vi "Compare Lists.vi"(4 "Right List":string, 5 "Left List":string, 6 "Compared Items in":string, 7 "Indent Level in":i32) -> (0 "Decicion Made ?":bool, 1 "In Right Order ?":bool, 2 "Compared Items out":string, 3 "Indent Level out":i32)   [LabVIEW 2020, in "AoC 2022.lvlib"]
uses:
  AoC 2022.lvlib
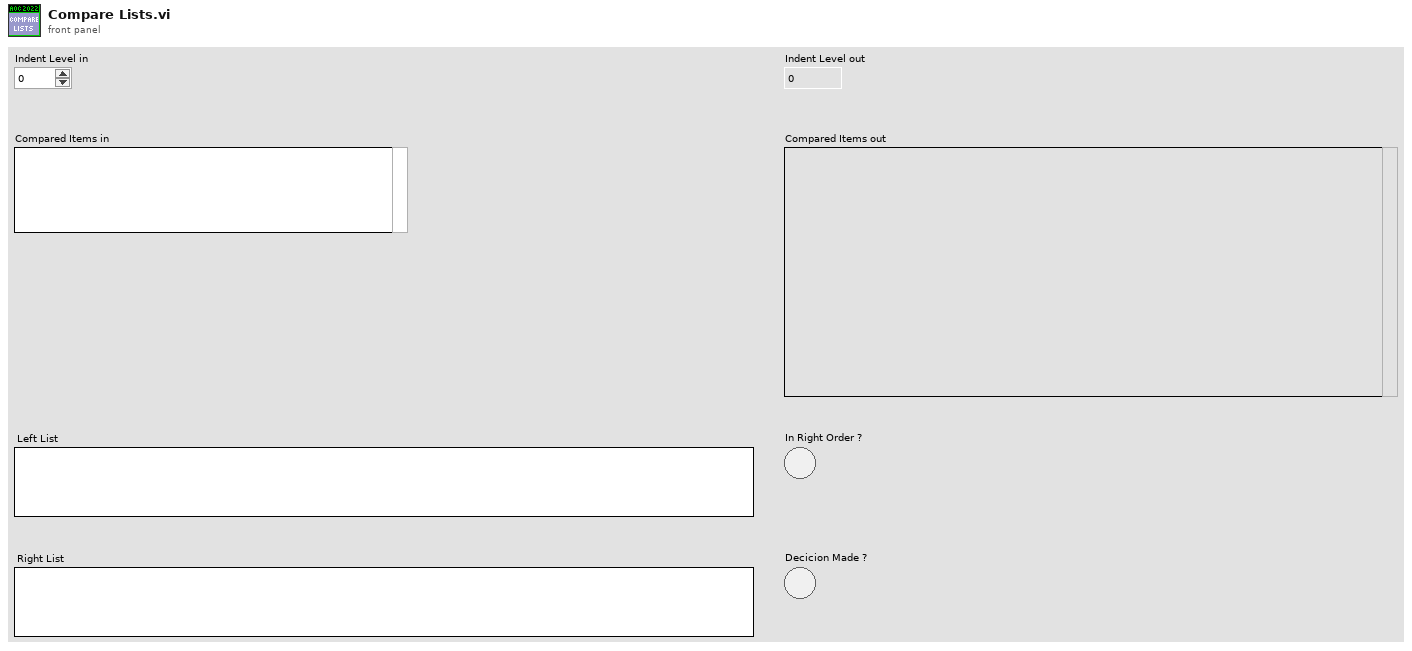
[diagram p1: front panel]
types:
  T1 = typedef "AoC 2022.lvlib/Item.ctl" = cluster{"Item Type":T2, "Item":string}
  T2 = typedef "AoC 2022.lvlib/Item Type.ctl" = enum16{"Integer", "List"}
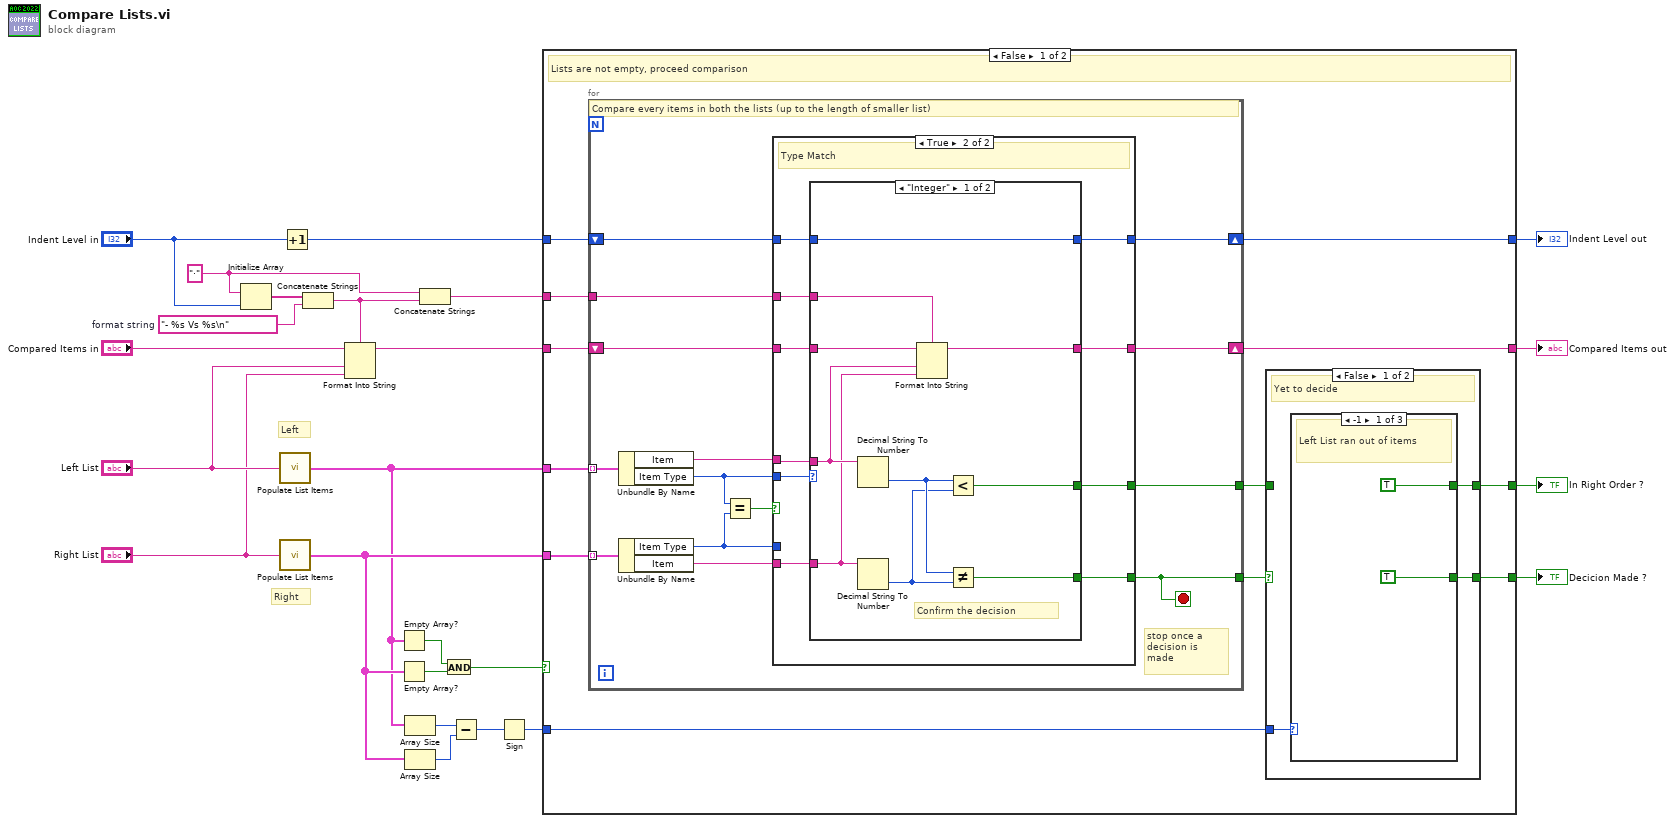
[diagram p0: block diagram]
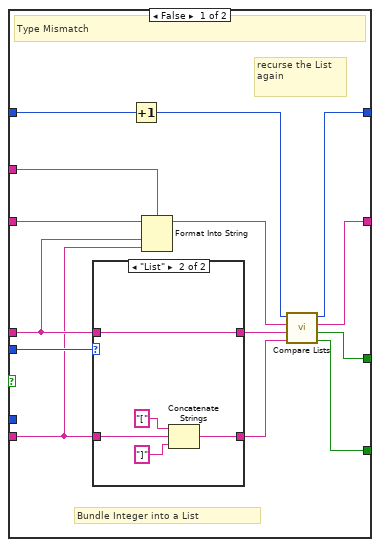
[diagram p2: hidden frame]
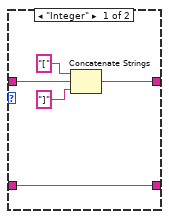
[diagram p3: hidden frame]
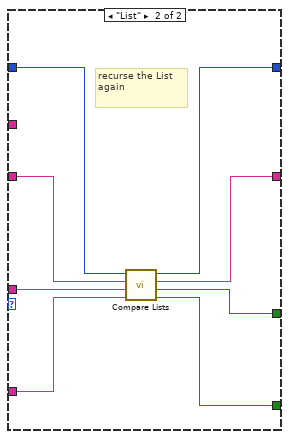
[diagram p4: hidden frame]
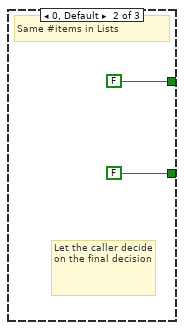
[diagram p5: hidden frame]
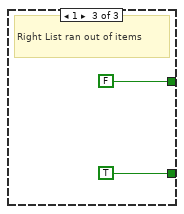
[diagram p6: hidden frame]
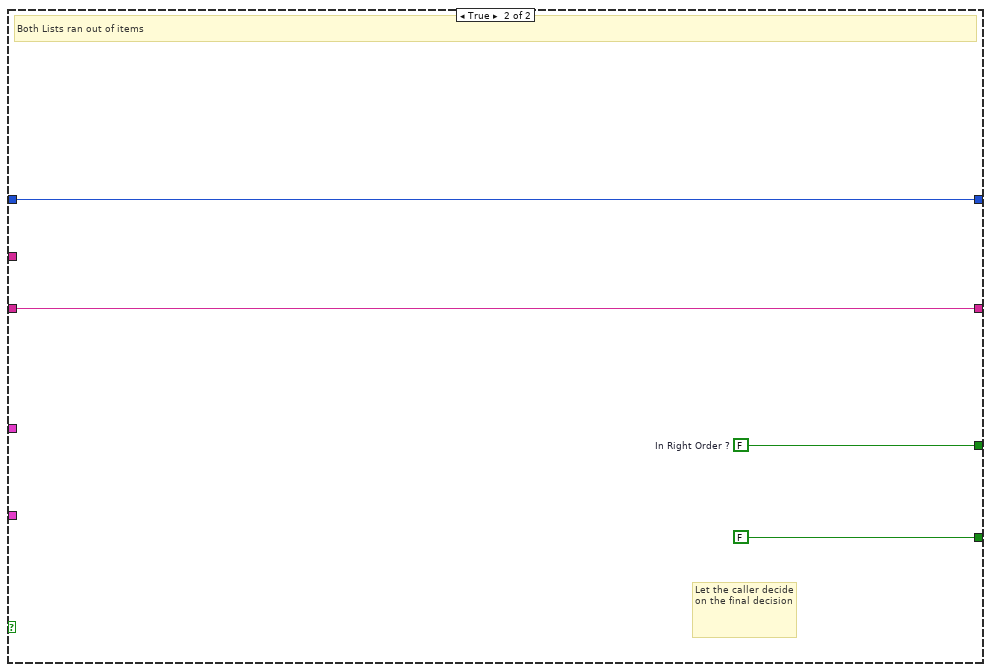
[diagram p8: hidden frame]
diagram:
  w11 = "·"
  w23 = "- %s Vs %s\n"  # format string
  # "Right"
  # "Left"
  n1 = Initialize Array(w11, "Indent Level in") -> (w20:string[])
  n2 = call "Populate List Items.vi"("List"="Left List") -> ("Items"=w8:T1[])
  n3 = call "Populate List Items.vi"("List"="Right List") -> ("Items"=w9:T1[])
  n4 = Increment(x="Indent Level in") -> (x+1=w10:i32)
  n5 = Concatenate Strings(w20, w23) -> (w13:string)
  n6 = Format Into String(format string=w13, initial string="Compared Items in", "Left List", "Right List") -> (resulting string=w16:string)  [unwired: 1 in, 1 out]
  n7 = Empty Array?(array=w8) -> (empty?=w6:bool)
  n8 = Empty Array?(array=w9) -> (empty?=w7:bool)
  n9 = Array Size(array=w8) -> (size(s)=w4:i32)
  n10 = Array Size(array=w9) -> (size(s)=w3:i32)
  n11 = Concatenate Strings(w11, w13) -> (w12:string)
  n12 = And(x=w6, y=w7) -> (x .and. y?=w5:bool)
  n13 = Subtract(x=w4, y=w3) -> (x-y=w2:i32)
  n14 = Sign(1:w2) -> (0:w1:i32)
  n15 = case shown="False" w5 {
    tunnel: w8 -> [w36 _]
    tunnel: [w25 FALSE] -> w24
    tunnel: [w35 w116] -> w22
    tunnel: [w27 w115] -> w21
    tunnel: [w34 w117] -> w18
    tunnel: w16 -> [w33 w116]
    tunnel: w12 -> [w32 _]
    tunnel: w10 -> [w31 w117]
    tunnel: w9 -> [w30 _]
    tunnel: w1 -> [w29 _]
    frame False {
      # "Lists are not empty, proceed comparison"
      n16 = for {
        tunnel: w36 -> [w50] mode=indexing
        tunnel: w30 -> [w49] mode=indexing
        tunnel: [w38] -> w26
        tunnel: [w37] -> w28
        tunnel: w32 -> [w41]
        shift-right: [w42] -> w35
        shift-left: w33 -> [w43]
        shift-right: [w39] -> w34
        shift-left: w31 -> [w40]
        stop <- w37 stop-if-true
        # "stop once a decision is made"
        # "Compare every items in both the lists (up to the length of smaller list)"
        n17 = Unbundle By Name(w50) -> ("Item"=w47:string, "Item Type"=w45:T2)
        n18 = Unbundle By Name(w49) -> ("Item Type"=w44:T2, "Item"=w46:string)
        n19 = Equal?(x=w45, y=w44) -> (x = y?=w48:bool)
        n20 = case shown="True" w48 {
          tunnel: w47 -> [w53 w83]
          tunnel: w46 -> [w52 w82]
          tunnel: w45 -> [w64 w84]
          tunnel: w44 -> [_ _]
          tunnel: [w63 w81] -> w38
          tunnel: [w62 w80] -> w37
          tunnel: [w61 w79] -> w42
          tunnel: w43 -> [w60 w78]
          tunnel: w41 -> [w59 w77]
          tunnel: w40 -> [w55 w76]
          tunnel: [w54 w75] -> w39
          frame False {
            # "recurse the List again"
            # "Bundle Integer into a List"
            # "Type Mismatch"
            n21 = case shown="\"List\"" w64 {
              tunnel: w53 -> [w69 w74]
              tunnel: [w66 w74] -> w58
              tunnel: [w65 w70] -> w57
              tunnel: w52 -> [w65 w71]
              frame "Integer" {
                n22 = Concatenate Strings("[", w69, "]") -> (w66:string)
              }
              frame "List" {
                n23 = Concatenate Strings("[", w71, "]") -> (w70:string)
              }
            }
            n24 = Increment(x=w55) -> (x+1=w51:i32)
            n25 = Format Into String(format string=w59, initial string=w60, w53, w52) -> (resulting string=w56:string)  [unwired: 1 in, 1 out]
            n26 = call "Compare Lists.vi"("Right List"=w57, "Left List"=w58, "Compared Items in"=w56, "Indent Level in"=w51) -> ("Decicion Made ?"=w62:bool, "In Right Order ?"=w63:bool, "Compared Items out"=w61:string, "Indent Level out"=w54:i32)
          }
          frame True {
            # "Type Match"
            n27 = case shown="\"Integer\"" w84 {
              tunnel: w83 -> [w91 w99]
              tunnel: w82 -> [w89 w98]
              tunnel: [w86 w102] -> w81
              tunnel: [w85 w101] -> w80
              tunnel: [w90 w100] -> w79
              tunnel: w78 -> [w88 w95]
              tunnel: w77 -> [w92 _]
              tunnel: w76 -> [w87 w97]
              tunnel: [w87 w96] -> w75
              frame "Integer" {
                # "Confirm the decision"
                n28 = Decimal String To Number(string=w91) -> (number=w94:i32)  [unwired: 2 in, 1 out]
                n29 = Decimal String To Number(string=w89) -> (number=w93:i32)  [unwired: 2 in, 1 out]
                n30 = Format Into String(format string=w92, initial string=w88, w91, w89) -> (resulting string=w90:string)  [unwired: 1 in, 1 out]
                n31 = Less?(x=w94, y=w93) -> (x < y?=w86:bool)
                n32 = Not Equal?(x=w94, y=w93) -> (x != y?=w85:bool)
              }
              frame "List" {
                # "recurse the List again"
                n33 = call "Compare Lists.vi"("Right List"=w98, "Left List"=w99, "Compared Items in"=w95, "Indent Level in"=w97) -> ("Decicion Made ?"=w101:bool, "In Right Order ?"=w102:bool, "Compared Items out"=w100:string, "Indent Level out"=w96:i32)
              }
            }
          }
        }
      }
      n34 = case shown="False" w28 {
        selector: w28 -> [_ w112]
        tunnel: w29 -> [w105 _]
        tunnel: [w104 w113] -> w27
        tunnel: w26 -> [_ w113]
        tunnel: [w103 w112] -> w25
        frame False {
          # "Yet to decide"
          n35 = case shown="-1" w105 {
            tunnel: [TRUE FALSE FALSE] -> w104
            tunnel: [TRUE FALSE TRUE] -> w103
            frame -1 {
              # "Left List ran out of items"
            }
            frame 0, Default {
              # "Let the caller decide on the final decision"
              # "Same #items in Lists"
            }
            frame 1 {
              # "Right List ran out of items"
            }
          }
        }
        frame True {
          # "Decision already made"
        }
      }
    }
    frame True {
      w115 = FALSE  # In Right Order ?
      # "Let the caller decide on the final decision"
      # "Both Lists ran out of items"
    }
  }
  "In Right Order ?" <- w21
  "Decicion Made ?" <- w24
  "Compared Items out" <- w22
  "Indent Level out" <- w18
